vi "WRP Check Analyzer Region.vi"(8 "error in (no error)":errorcluster) -> (0 "error out":errorcluster, 1 "time_ms":dbl, 2 "steps":i32, 3 "analyzerRegion":T1, 4 "function return":i32, 5 "energyStep":dbl)   [LabVIEW 2018, in "SesWrapper.lvlib"]
doc: "int STDCALL WRP_CheckAnalyzerRegion(AnalyzerRegion *analyzerRegion, int *steps, double *time_ms, double *energyStep);"
uses:
  SesWrapper.lvlib
  build/Debug/SESWrapper.dll
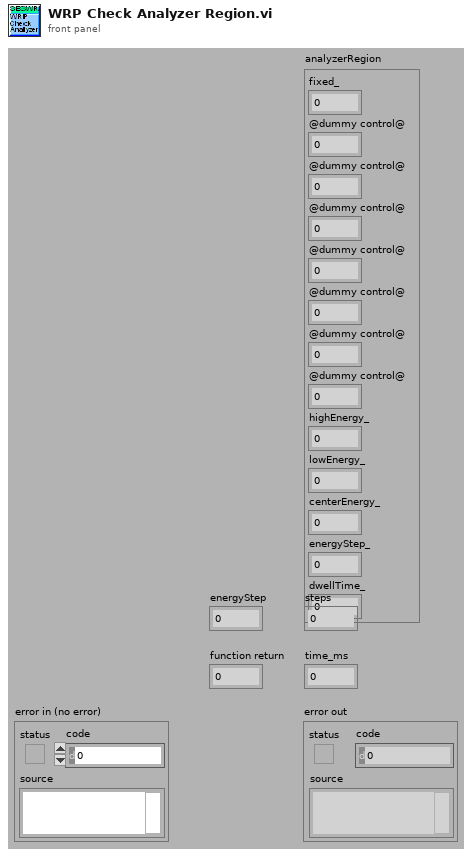
[diagram p1: front panel]
types:
  T1 = cluster{"fixed_":u8, "@dummy control@":i8, "@dummy control@":i8, "@dummy control@":i8, "@dummy control@":i8, "@dummy control@":i8, "@dummy control@":i8, "@dummy control@":i8, "highEnergy_":dbl, "lowEnergy_":dbl, "centerEnergy_":dbl, "energyStep_":dbl, "dwellTime_":i32}
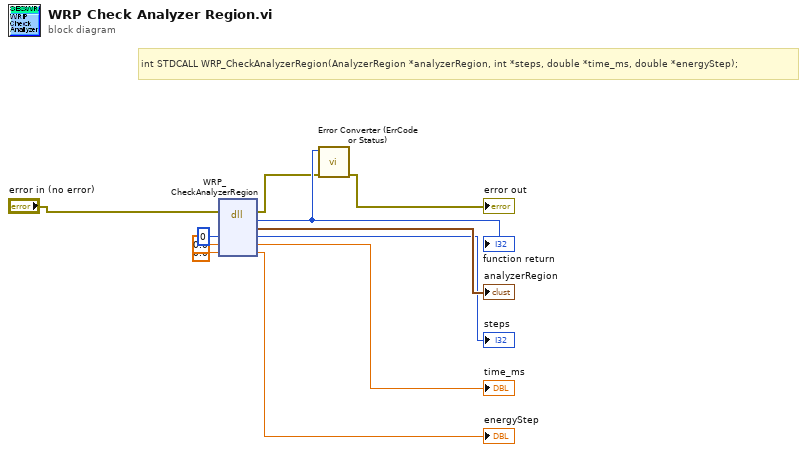
[diagram p0: block diagram]
diagram:
  # "int STDCALL WRP_CheckAnalyzerRegion(AnalyzerRegion *analyzerRegion, int *steps, double *time_ms, double *energyStep);"
  n1 = dll-call lib="C:/Development/svn/seswrapper-lib/build/Debug/SESWrapper.*" fn="WRP_CheckAnalyzerRegion"(error in="error in (no error)", "steps"=0, "time_ms"=0.0, "energyStep"=0.0) -> (error out=w2:errorcluster, w11:i32, "analyzerRegion"=→"analyzerRegion":T1, "steps"=→"steps":i32, "time_ms"=→"time_ms":dbl, "energyStep"=→"energyStep":dbl)  [unwired: 3 in, 1 out]
  "function return" <- w11
  n2 = call "Error Converter (ErrCode or Status).vi"("error in (no error)"=w2, "error code"=w11) -> ("error out"=→"error out":errorcluster)  [unwired: 9 in]
